vi "main(Test DQMH modules).vi"() -> ()   [LabVIEW 2018, in "Application.lvlib"]
uses:
  Application.lvlib
  eMIC response.ctl
  type defs/HW config.ctl
  eMICs Cluster.ctl
  SubVIs/App state data.ctl
  SubVIs/Trigger cluster.ctl
  SubVIs/FGV DRV data.ctl
  type defs/DMM all config cluster.ctl
  type defs/DMM config cluster.ctl
  SubVIs/DUT data Mode.ctl
  Instrument Drivers/LV_driver_MBrelay/type defs/FGV enum.ctl
  SubVIs/Step data.ctl
  DRV cluster 2.ctl
  <vilib>/ErrorRing/Error Ring.xnode
  Switches Module/MB switches Module.lvlib
  MB 01 switches Module/MB 01 switches Module.lvlib
  DMM Module/DMM Module.lvlib
  v2_CE14/CE14_v2.lvlib
  Instrument Drivers/LV_driver_MBrelay/MB Relay.lvlib
panel:
  out "List of Actions":string[](array[string])
  out "1":u32(colorbox)
  out "elapsed Time":string
  out "#DRV":string
  out "Report file Name":string
  in  "RE_Test":bool caption="Again"
  in  "wait for (ms)":u32=3000
  in  "Log report":bool
  in  "DRV number":u8=1 max=60
  in  "Test Single DRV":bool
  out "DUT Name":string
  out "SAP ID":string
  out "Progress Status":string
  in  "Auto/Man":bool
  out "DC Measure Completed":bool caption="DC Completed"
  in  "Test Channel 10":bool
  in  "Test Channel 9":bool
  in  "Test Channel 8":bool
  in  "Test Channel 7":bool
  in  "Test Channel 6":bool
  in  "Test Channel 5":bool
  in  "Test Channel 4":bool
  in  "Test Channel 3":bool
  in  "Test Channel 2":bool
  in  "Test Channel 1":bool
  in  "Shorted Circuits Test":bool
  out "CE14  Module did it":bool[](array[boolean])
  out "Inst. 9":bool
  in  "Exit":bool
  out "Inst. 8":bool
  out "Inst. 7":bool
  out "Inst. 6":bool
  out "Inst. 5":bool
  out "Inst. 4":bool
  out "Inst. 3":bool
  out "Inst. 2":bool
  out "Inst. 1":bool
  out "new Trigger?":bool
  out "last Trigger?":bool
  out "error out":errorcluster
  out "State log":string
  out "AC  Completed":bool caption="AC Completed"
  in  "Select CE14 eMIC Module Instance":i32(ring)=-1 items=["All"=-1, "1"=1, "2"=2, "3"=3, "4"=4, "5"=5, "6"=6]
  out "New board?":bool
  in  "Test":bool caption="Again"
  out "DRV 61":u32(colorbox)
  in  "Settings":bool
  in  "VIEW":bool caption="Again"
  out "DRV 60":u32(colorbox) caption="60"
  out "DRV 59":u32(colorbox) caption="59"
  out "DRV 58":u32(colorbox) caption="58"
  out "DRV 57":u32(colorbox) caption="57"
  out "DRV 56":u32(colorbox) caption="56"
  out "DRV 55":u32(colorbox) caption="55"
  out "DRV 54":u32(colorbox) caption="54"
  out "DRV 53":u32(colorbox) caption="53"
  out "DRV 52":u32(colorbox) caption="52"
  out "DRV 51":u32(colorbox) caption="51"
  out "DRV 50":u32(colorbox) caption="50"
  out "DRV 49":u32(colorbox) caption="49"
  out "DRV 48":u32(colorbox) caption="48"
  out "DRV 47":u32(colorbox) caption="47"
  out "DRV 46":u32(colorbox) caption="46"
  out "DRV 45":u32(colorbox) caption="45"
  out "DRV 44":u32(colorbox) caption="44"
  out "DRV 43":u32(colorbox) caption="43"
  out "DRV 42":u32(colorbox) caption="42"
  out "DRV 41":u32(colorbox) caption="41"
  out "DRV 40":u32(colorbox) caption="40"
  out "DRV 39":u32(colorbox) caption="39"
  out "DRV 38":u32(colorbox) caption="38"
  out "DRV 37":u32(colorbox) caption="37"
  out "DRV 36":u32(colorbox) caption="36"
  out "DRV 35":u32(colorbox) caption="35"
  out "DRV 34":u32(colorbox) caption="34"
  out "DRV 33":u32(colorbox) caption="33"
  out "DRV 32":u32(colorbox) caption="32"
  out "DRV 31":u32(colorbox) caption="31"
  out "DRV 30":u32(colorbox) caption="30"
  out "DRV 29":u32(colorbox) caption="29"
  out "DRV 28":u32(colorbox) caption="28"
  out "DRV 27":u32(colorbox) caption="27"
  out "DRV 26":u32(colorbox) caption="26"
  out "DRV 25":u32(colorbox) caption="25"
  out "DRV 24":u32(colorbox) caption="24"
  out "DRV 23":u32(colorbox) caption="23"
  out "DRV 22":u32(colorbox) caption="22"
  out "DRV 21":u32(colorbox) caption="21"
  out "DRV 20":u32(colorbox) caption="20"
  out "DRV 19":u32(colorbox) caption="19"
  out "DRV 18":u32(colorbox) caption="18"
  out "DRV 17":u32(colorbox) caption="17"
  out "DRV 16":u32(colorbox) caption="16"
  out "DRV 15":u32(colorbox) caption="15"
  out "DRV 14":u32(colorbox) caption="14"
  out "DRV 13":u32(colorbox) caption="13"
  out "DRV 12":u32(colorbox) caption="12"
  out "DRV 11":u32(colorbox) caption="11"
  out "DRV 10":u32(colorbox) caption="10"
  out "DRV 9":u32(colorbox) caption="9"
  out "DRV 8":u32(colorbox) caption="8"
  out "DRV 7":u32(colorbox) caption="7"
  out "DRV 6":u32(colorbox) caption="6"
  out "DRV 5":u32(colorbox) caption="5"
  out "DRV 4":u32(colorbox) caption="4"
  out "DRV 3":u32(colorbox) caption="3"
  out "DRV 2":u32(colorbox) caption="2"
  out "DRV 1":u32(colorbox) caption="1"
  out "version":string caption="Version"
  out "Module ID":i32
  in  "Tab Control":T1(tab)
  out "Short DRV":bool[][](array[boolean])
  in  "Mux 10-1":bool
  in  "mux 6-1":bool
  in  "Read Optos":bool
  in  "Select DMM's Current Input":bool
  in  "mux2-1(DMM I) encode":enum16{"DMM I (0.5)", "DMM I (12)"}(ring)
  in  "mux 6-1 data":T2(ring)
  in  "mux 10-1 data":T3(ring)
  in  "set value":bool
  in  "Set trigger value":bool
  out "trigger Value":bool
  in  "Read trigger":bool
  in  "Reset JIG":bool
  in  "eMIC":bool
  in  "DEMUX 1-10":bool
  in  "TurnON/OFF +5V":bool
  in  "5V Value":bool
  in  "demux1_10(x6)_encode":T4(ring)
  in  "eMIC 6 values":bool[](array[boolean])=[FALSE, FALSE, FALSE, FALSE, FALSE, FALSE]
  in  "DMM query":bool
  in  "connect DMM":bool
  in  "DMM read dual value":bool
  in  "config DMM":bool
  in  "Detector Rate":u8(ring)=2 items=["SLOW", "MID", "FAST"]
  in  "DCI range":dbl=0.5
  in  "DCV range":dbl=1000.0
  out "DCV(Volts)":dbl
  out "DCI(mA)":dbl
  out "DMM func?":string
  out "DMM range?":string
  in  "request AC-all":bool
  in  "Open COM eMIC":bool
  in  "check connected":bool
  out "eMIC 1":T5
  out "eMIC 2":T5
  out "eMIC 3":T5
  out "eMIC 4":T5
  out "eMIC 5":T5
  out "eMIC 6":T5
  out "EMIC connected":bool[](array[boolean])
  out "AC switches Module":bool
  out "DC Measure Module":bool
  out "DC Switches Module":bool
  out "AC Measure Module":bool
  # "HV-60D: ON-LINE TESTER FOR LED POWER DRIVER"
  # "60"
  # "6"
  # "12"
  # "18"
  # "24"
  # "30"
  # "36"
  # "42"
  # "48"
  # "54"
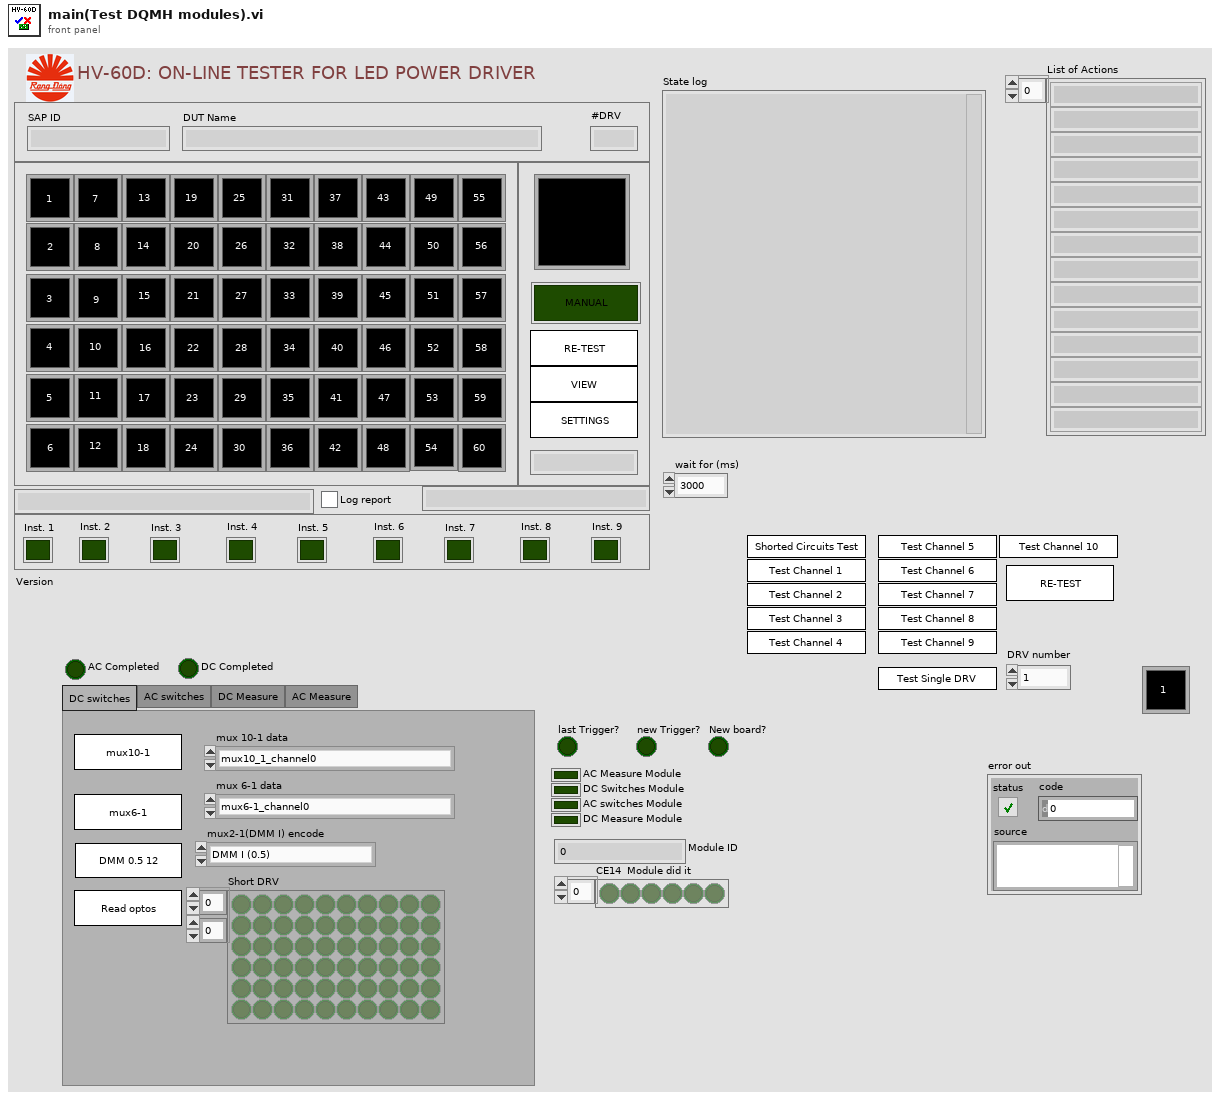
[diagram p1: front panel]
types:
  T1 = enum32{"DC switches", "AC switches", "DC Measure", "AC Measure"}
  T2 = enum16{"mux6-1_channel0", "mux6_1_channel1_0", "mux6_1_channel1_1", "mux6-1_channel1_2", "mux6_1_channel1_3", "mux6_1_channel2_0", "mux6_1_channel2_1", "mux6_1_channel2_2", "mux6_1_channel2_3", "mux6_1_channel3_0", "mux6_1_channel3_1", "mux6_1_channel3_2", "mux6_1_channel3_3", "mux6_1_channel4_0", "mux6_1_channel4_1", "mux6_1_channel4_2", "mux6_1_channel4_3", "mux6_1_channel5_0", "mux6_1_channel5_1", "mux6_1_channel5_2", "mux6_1_channel5_3", "mux6_1_channel6_0", "mux6_1_channel6_1", "mux6_1_channel6_2", "mux6_1_channel6_3"}
  T3 = enum16{"mux10_1_channel0", "mux10_1_channel1", "mux10_1_channel2", "mux10_1_channel3", "mux10_1_channel4", "mux10_1_channel5", "mux10_1_channel6", "mux10_1_channel7", "mux10_1_channel8", "mux10_1_channel9", "mux10_1_channel10"}
  T4 = enum16{"demux1_10_channel0", "demux1_10_channel1", "demux1_10_channel2", "demux1_10_channel3", "demux1_10_channel4", "demux1_10_channel5", "demux1_10_channel6", "demux1_10_channel7", "demux1_10_channel8", "demux1_10_channel9", "demux1_10_channel10"}
  T5 = typedef "Application.lvlib/eMIC response.ctl" = cluster{"ACV":dbl, "ACI":dbl, "pF":dbl, "kW":dbl, "Freq":dbl, "kvar":dbl}
  T6 = typedef "Application.lvlib/eMICs Cluster.ctl" = cluster{"eMIC 1":T5, "eMIC 2":T5, "eMIC 3":T5, "eMIC 4":T5, "eMIC 5":T5, "eMIC 6":T5}
  T7 = typedef "Application.lvlib/HW config.ctl" = cluster{"DMM":string, "mux":string, "demux":string, "eMIC1":string, "eMIC2":string, "eMIC3":string, "eMIC4":string, "eMIC5":string, "eMIC6":string}
  T8 = typedef "Application.lvlib/Trigger cluster.ctl" = cluster{"new board?":bool, "new trigger":bool, "last trigger":bool}
  T9 = typedef "Application.lvlib/App state data.ctl" = cluster{"command":string, "data":variant}
  T10 = typedef "CE14_v2.lvlib/Broadcast Events--cluster.ctl" = cluster{"Module Did Init":refnum<user-event>, "Status Updated":refnum<user-event>, "Error Reported":refnum<user-event>, "Module Did Stop":refnum<user-event>, "Update Module Execution Status":refnum<user-event>, "CE14 response data":refnum<user-event>}
  T11 = typedef "MB switches Module.lvlib/Broadcast Events--cluster.ctl" = cluster{"Module Did Init":refnum<user-event>, "Status Updated":refnum<user-event>, "Error Reported":refnum<user-event>, "Module Did Stop":refnum<user-event>, "Update Module Execution Status":refnum<user-event>}
  T12 = typedef "MB 01 switches Module.lvlib/Broadcast Events--cluster.ctl" = cluster{"Module Did Init":refnum<user-event>, "Status Updated":refnum<user-event>, "Error Reported":refnum<user-event>, "Module Did Stop":refnum<user-event>, "Update Module Execution Status":refnum<user-event>}
  T13 = typedef "DMM Module.lvlib/Broadcast Events--cluster.ctl" = cluster{"Module Did Init":refnum<user-event>, "Status Updated":refnum<user-event>, "Error Reported":refnum<user-event>, "Module Did Stop":refnum<user-event>, "Update Module Execution Status":refnum<user-event>}
  T14 = enum16{"open", "replace", "create", "open or create", "replace or create", "replace or create with confirmation"}
  T15 = typedef "Application.lvlib/DRV cluster 2.ctl" = cluster{"Shorted Circuit":bool, "AC voltage(volts)":dbl, "AC Current (mA)":dbl, "AC kW (W)":dbl, "AC pF ":dbl, "DC Voltage (Volts)":dbl, "DC Current (mA)":dbl, "DC kW (W)":dbl, "DRV Fail/Pass (T)":bool, "efficient (%)":dbl}
  T16 = typedef "Application.lvlib/DRV stand.ctl" = cluster{"SAP ID":string, "Name":string, "AC characteristics":cluster{"Voltage":cluster{"Min":dbl, "Max":dbl}, "Current":cluster{"Min":dbl, "Max":dbl}, "kW":cluster{"Min":dbl, "Max":dbl}, "PF":cluster{"Min":dbl, "Max":dbl}}, "DC characteristics":cluster{"Voltage":cluster{"Min":dbl, "Max":dbl}, "Current":cluster{"Min":dbl, "Max":dbl}, "Effect":cluster{"Min":dbl, "Max":dbl}}, "Sub-Test":cluster{"ACV":bool, "ACI":bool, "kW":bool, "PF":bool, "DCV":bool, "DCI":bool, "efficiency":bool}}
  T17 = enum32{"Invalid", "Standard", "Closed", "Hidden", "Minimized", "Maximized"}
  T18 = typedef "Application.lvlib/FGV DRV data.ctl" = enum16{"Init", "Write", "Read", "Process"}
  T19 = typedef "Application.lvlib/DMM all config cluster.ctl" = cluster{"DMM config cluster":T20, "mux2-1(DMM I) encode":enum16{"DMM I (0.5)", "DMM I (12)"}}
  T20 = typedef "Application.lvlib/DMM config cluster.ctl" = cluster{"DCV range":dbl, "DCI range":dbl, "Detector Rate":u8}
  T21 = typedef "Application.lvlib/DUT data Mode.ctl" = enum16{"range Limit", "Short Circuits", "AC parameter", "AC parameter 1", "DC parameter"}
  T22 = typedef "MB Relay.lvlib/FGV enum.ctl" = enum16{"Write", "Init FGV", "Read", "All OFF", "All ON"}
  T23 = typedef "CE14_eMIC.lvlib/CE14.data.ctl" = cluster{"string":string, "float":dbl, "Name":string}
  T24 = typedef "Application.lvlib/Step data.ctl" = cluster{"command":string, "Data":variant}
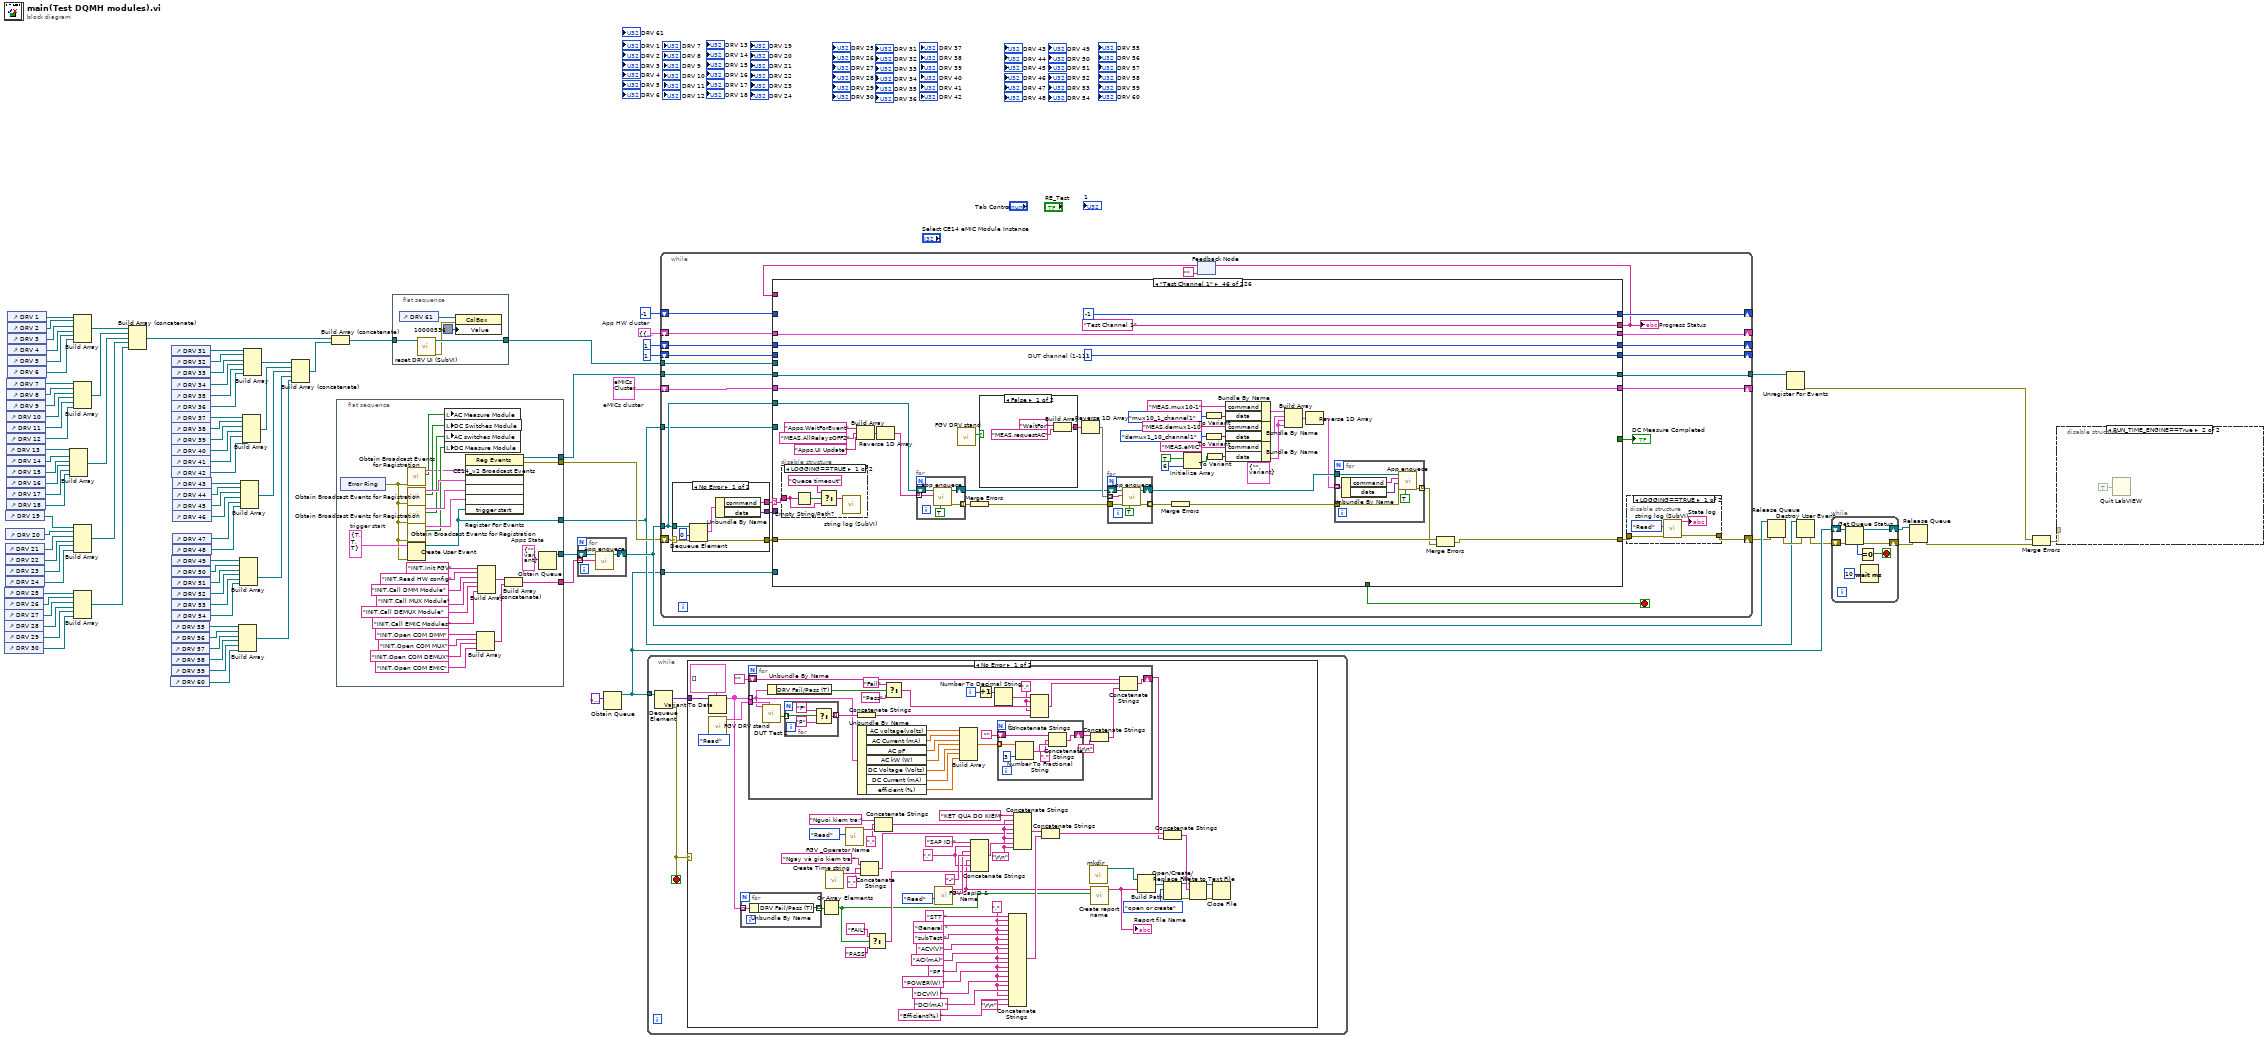
[diagram p0: block diagram]
diagram:
  w88 = T6 {"eMIC 1"={"ACV"=0.0, "ACI"=0.0, "pF"=0.0, "kW"=0.0, "Freq"=0.0, "kvar"=0.0}, "eMIC 2"={"ACV"=0.0, "ACI"=0.0, "pF"=0.0, "kW"=0.0, "Freq"=0.0, "kvar"=0.0}, "eMIC 3"={"ACV"=0.0, "ACI"=0.0, "pF"=0.0, "kW"=0.0, "Freq"=0.0, "kvar"=0.0}, "eMIC 4"={"ACV"=0.0, "ACI"=0.0, "pF"=0.0, "kW"=0.0, "Freq"=0.0, "kvar"=0.0}, "eMIC 5"={"ACV"=0.0, "ACI"=0.0, "pF"=0.0, "kW"=0.0, "Freq"=0.0, "kvar"=0.0}, "eMIC 6"={"ACV"=0.0, "ACI"=0.0, "pF"=0.0, "kW"=0.0, "Freq"=0.0, "kvar"=0.0}}  # eMICs cluster
  w93 = cluster{"HW config 2":T7} {"HW config 2"={"DMM"="COM15", "mux"="COM11", "demux"="COM16", "eMIC1"="COM13", "eMIC2"="COM6", "eMIC3"="COM9", "eMIC4"="COM10", "eMIC5"="COM12", "eMIC6"="COM11"}}  # App HW cluster
  n1 = control-ref of="DRV 25"() -> (w58:refnum<vi>)
  n2 = control-ref of="DRV 26"() -> (w59:refnum<vi>)
  n3 = control-ref of="DRV 27"() -> (w60:refnum<vi>)
  n4 = control-ref of="DRV 28"() -> (w61:refnum<vi>)
  n5 = control-ref of="DRV 29"() -> (w62:refnum<vi>)
  n6 = control-ref of="DRV 30"() -> (w63:refnum<vi>)
  n7 = control-ref of="DRV 21"() -> (w67:refnum<vi>)
  n8 = control-ref of="DRV 22"() -> (w66:refnum<vi>)
  n9 = control-ref of="DRV 23"() -> (w65:refnum<vi>)
  n10 = control-ref of="DRV 24"() -> (w64:refnum<vi>)
  n11 = control-ref of="DRV 19"() -> (w69:refnum<vi>)
  n12 = control-ref of="DRV 20"() -> (w68:refnum<vi>)
  n13 = control-ref of="DRV 13"() -> (w75:refnum<vi>)
  n14 = control-ref of="DRV 7"() -> (w81:refnum<vi>)
  n15 = control-ref of="DRV 8"() -> (w80:refnum<vi>)
  n16 = control-ref of="DRV 9"() -> (w79:refnum<vi>)
  n17 = control-ref of="DRV 10"() -> (w78:refnum<vi>)
  n18 = control-ref of="DRV 11"() -> (w77:refnum<vi>)
  n19 = control-ref of="DRV 12"() -> (w76:refnum<vi>)
  n20 = control-ref of="DRV 14"() -> (w74:refnum<vi>)
  n21 = control-ref of="DRV 15"() -> (w73:refnum<vi>)
  n22 = control-ref of="DRV 16"() -> (w72:refnum<vi>)
  n23 = control-ref of="DRV 17"() -> (w71:refnum<vi>)
  n24 = control-ref of="DRV 18"() -> (w70:refnum<vi>)
  n25 = control-ref of="DRV 1"() -> (w87:refnum<vi>)
  n26 = control-ref of="DRV 2"() -> (w86:refnum<vi>)
  n27 = control-ref of="DRV 3"() -> (w85:refnum<vi>)
  n28 = control-ref of="DRV 4"() -> (w84:refnum<vi>)
  n29 = control-ref of="DRV 5"() -> (w83:refnum<vi>)
  n30 = control-ref of="DRV 6"() -> (w82:refnum<vi>)
  n31 = Build Array(w75, w74, w73, w72, w71, w70) -> (w55:refnum<vi>[])
  n32 = Build Array(w87, w86, w85, w84, w83, w82) -> (w57:refnum<vi>[])
  n33 = Build Array(w69, w68, w67, w66, w65, w64) -> (w54:refnum<vi>[])
  n34 = Build Array(w58, w59, w60, w61, w62, w63) -> (w53:refnum<vi>[])
  n35 = Build Array(w81, w80, w79, w78, w77, w76) -> (w56:refnum<vi>[])
  n36 = Build Array (concatenate)(w57, w56, w55, w54, w53) -> (w17:refnum<vi>[])
  n37 = control-ref of="DRV 60"() -> (w28:refnum<vi>)
  n38 = control-ref of="DRV 55"() -> (w23:refnum<vi>)
  n39 = control-ref of="DRV 56"() -> (w24:refnum<vi>)
  n40 = control-ref of="DRV 57"() -> (w25:refnum<vi>)
  n41 = control-ref of="DRV 58"() -> (w26:refnum<vi>)
  n42 = control-ref of="DRV 59"() -> (w27:refnum<vi>)
  n43 = control-ref of="DRV 31"() -> (w47:refnum<vi>)
  n44 = control-ref of="DRV 32"() -> (w48:refnum<vi>)
  n45 = control-ref of="DRV 33"() -> (w49:refnum<vi>)
  n46 = control-ref of="DRV 34"() -> (w50:refnum<vi>)
  n47 = control-ref of="DRV 35"() -> (w51:refnum<vi>)
  n48 = control-ref of="DRV 36"() -> (w52:refnum<vi>)
  n49 = control-ref of="DRV 37"() -> (w46:refnum<vi>)
  n50 = control-ref of="DRV 38"() -> (w45:refnum<vi>)
  n51 = control-ref of="DRV 39"() -> (w44:refnum<vi>)
  n52 = control-ref of="DRV 40"() -> (w43:refnum<vi>)
  n53 = control-ref of="DRV 41"() -> (w42:refnum<vi>)
  n54 = control-ref of="DRV 42"() -> (w41:refnum<vi>)
  n55 = control-ref of="DRV 49"() -> (w34:refnum<vi>)
  n56 = control-ref of="DRV 50"() -> (w33:refnum<vi>)
  n57 = control-ref of="DRV 51"() -> (w32:refnum<vi>)
  n58 = control-ref of="DRV 52"() -> (w31:refnum<vi>)
  n59 = control-ref of="DRV 53"() -> (w30:refnum<vi>)
  n60 = control-ref of="DRV 54"() -> (w29:refnum<vi>)
  n61 = control-ref of="DRV 43"() -> (w35:refnum<vi>)
  n62 = control-ref of="DRV 44"() -> (w36:refnum<vi>)
  n63 = control-ref of="DRV 45"() -> (w37:refnum<vi>)
  n64 = control-ref of="DRV 46"() -> (w38:refnum<vi>)
  n65 = control-ref of="DRV 47"() -> (w39:refnum<vi>)
  n66 = control-ref of="DRV 48"() -> (w40:refnum<vi>)
  n67 = Build Array(w23, w24, w25, w26, w27, w28) -> (w18:refnum<vi>[])
  n68 = Build Array(w34, w33, w32, w31, w30, w29) -> (w19:refnum<vi>[])
  n69 = Build Array(w35, w36, w37, w38, w39, w40) -> (w20:refnum<vi>[])
  n70 = Build Array(w46, w45, w44, w43, w42, w41) -> (w21:refnum<vi>[])
  n71 = Build Array(w47, w48, w49, w50, w51, w52) -> (w22:refnum<vi>[])
  n72 = Build Array (concatenate)(w22, w21, w20, w19, w18) -> (w16:refnum<vi>[])
  n73 = Build Array (concatenate)(w17, w16) -> (w14:refnum<vi>[])
  n74 = flat-sequence {
    tunnel: [w118] -> w95
    tunnel: [w117] -> w92
    tunnel: [w116] -> w91
    tunnel: [w115] -> w15
    tunnel: [w110] -> w7
    frame #0 {
      w111 = T8 {"new board?"=TRUE, "new trigger"=TRUE, "last trigger"=TRUE}  # trigger start
      w112 = T9 {"command"="", "data"=variant}  # Apps State
      n75 = xnode "Error Ring"() -> ("error out"=w109:errorcluster)
      n76 = call "Obtain Broadcast Events for Registration.vi"("error in (no error)"=w109) -> ("Already running?"=w113:bool, "CE14_v2 Broadcast Events"=w114:T10)  [unwired: 8 in, 1 out]
      n77 = call "Obtain Broadcast Events for Registration.vi"("error in (no error)"=w109) -> ("Already running?"=w121:bool, "Switches Module Broadcast Events"=w124:T11)  [unwired: 8 in, 1 out]
      n78 = call "Obtain Broadcast Events for Registration.vi"("error in (no error)"=w109) -> ("Already running?"=w120:bool, "MB 01 switches Module Broadcast Events"=w123:T12)  [unwired: 8 in, 1 out]
      n79 = call "Obtain Broadcast Events for Registration.vi"("error in (no error)"=w109) -> ("Already running?"=w119:bool, "DMM Module Broadcast Events"=w122:T13)  [unwired: 8 in, 1 out]
      n80 = Create User Event(user event datatype=w111, error in=w109) -> (user event=w110:refnum<user-event>)  [unwired: 1 out]
      n81 = local write "AC Measure Module"(w113) -> ()
      n82 = local write "DC Switches Module"(w121) -> ()
      n83 = local write "AC switches Module"(w120) -> ()
      n84 = local write "DC Measure Module"(w119) -> ()
      n85 = register-events(w114, w124, w123, w122, w110) -> (reference out=w118:refnum<event-registration>, error out=w115:errorcluster)  [unwired: 2 in]
      n86 = Build Array("INIT.Open COM DMM", "INIT.Open COM MUX", "INIT.Open COM DEMUX", "INIT.Open COM EMIC") -> (w106:string[])
      n87 = Build Array("INIT.Init FGV", "INIT.Read HW config", "INIT.Call DMM Module", "INIT.Call MUX Module", "INIT.Call DEMUX Module", "INIT.Call EMIC Modules") -> (w107:string[])
      n88 = Build Array (concatenate)(w107, w106) -> (w116:string[])
      n89 = Obtain Queue(element data type=w112) -> (queue out=w117:refnum<queue>)  [unwired: 4 in, 2 out]
    }
  }
  n90 = flat-sequence {
    tunnel: w14 -> [w130]
    tunnel: [w129] -> w13
    frame #0 {
      n91 = control-ref of="DRV 61"() -> (w126:refnum<vi>)
      n92 = call "reset DRV UI (SubVI).vi"("Ref  in"=w130) -> ("error out"=w127:errorcluster, "Ref out"=w129:refnum<vi>[])  [unwired: 9 in]
      n93 = property class="ColBox"(reference=w126, error in=w127, "Value"=u32 10000536 ("DRV 1")) -> ()  [unwired: 2 out]
    }
  }
  n94 = for {
    tunnel: w91 -> [w133] mode=indexing
    shift-right: [w131] -> w90
    shift-left: w92 -> [w132]
    n95 = call "App enquece.vi"("command"=w133, "queue in"=w132) -> ("Queue out"=w131:refnum<queue>)  [unwired: 8 in, 1 out]
  }
  n96 = Obtain Queue(element data type=variant) -> (queue out=w5:refnum<queue>)  [unwired: 4 in, 2 out]
  n97 = while {
    tunnel: w5 -> [w136]
    stop <- w134 stop-if-true
    n98 = Dequeue Element(queue=w136) -> (element=w135:variant, error out=w134:errorcluster)  [unwired: 2 in, 2 out]
    n99 = case shown="No Error" w134 {
      tunnel: w135 -> [w189 _]
      frame No Error {
        w156 = ","
        w140 = ","
        w163 = "\r\n"
        n100 = Variant To Data(type=T15[] [] ("60 DRV data"), Variant=w189) -> (data=w144:T15[])  [unwired: 1 in, 1 out]
        n101 = call "FGV DRV stand.vi"("Enum(read)"=enum16{"Write", "Read"}."Read" ("Enum 2")) -> ("DRV stand out"=w187:T16)  [unwired: 9 in, 1 out]
        n102 = for {
          tunnel: w144 -> [w192] mode=indexing
          tunnel: [w191] -> w141 mode=indexing
          n103 = Unbundle By Name(w192) -> ("DRV Fail/Pass (T)"=w191:bool)
        }
        n104 = for {
          tunnel: w144 -> [w209] mode=indexing
          tunnel: w187 -> [w220]
          shift-right: [w197] -> w165
          shift-left: "" -> [w196]
          i -> [w214]
          w193 = ","
          n105 = call "DUT Test 2.vi"("DRV stand"=w220, "DRV data"=w209) -> ("actual subtest"=w216:bool[])  [unwired: 6 in, 3 out]
          n106 = Unbundle By Name(w209) -> ("DRV Fail/Pass (T)"=w219:bool)
          n107 = for {
            tunnel: w216 -> [w229] mode=indexing
            tunnel: [w228] -> w215 mode=indexing
            n108 = Select(t="F", s=w229, f="P") -> (s? t:f=w228:string)
          }
          n109 = Concatenate Strings(w215) -> (w210:string)
          n110 = Unbundle By Name(w209) -> ("AC voltage(volts)"=w208:dbl, "AC Current (mA)"=w207:dbl, "AC pF"=w206:dbl, "AC kW (W)"=w205:dbl, "DC Voltage (Volts)"=w204:dbl, "DC Current (mA)"=w203:dbl, "efficient (%)"=w202:dbl)
          n111 = Select(t="Fail", s=w219, f="Pass") -> (s? t:f=w211:string)
          n112 = Build Array(w208, w207, w206, w205, w204, w203, w202) -> (w201:dbl[])
          n113 = Increment(x=w214) -> (x+1=w213:i32)
          n114 = Number To Decimal String(number=w213) -> (decimal integer string=w212:string)  [unwired: 1 in]
          n115 = for {
            tunnel: w201 -> [w226] mode=indexing
            shift-right: [w223] -> w199
            shift-left: "" -> [w224]
            n116 = Number To Fractional String(number=w226, precision (6)=i16 3) -> (F-format string=w222:string)  [unwired: 2 in]
            n117 = Concatenate Strings(w224, ",", w222) -> (w223:string)
          }
          n118 = Concatenate Strings(w212, w193, w211, w193, w210) -> (w195:string)
          n119 = Concatenate Strings(w199, "\r\n") -> (w194:string)
          n120 = Concatenate Strings(w196, w195, w194) -> (w197:string)
        }
        n121 = Or Array Elements(Boolean array=w141) -> (logical OR=w137:bool)
        n122 = call "Create Time string.vi"() -> ("Timestr"=w161:string)  [unwired: 10 in, 1 out]
        n123 = call "FGV _Operator Name.vi"("Enum"=enum16{"Write", "Read"}."Read") -> ("Operator Name out"=w185:string)  [unwired: 10 in]
        n124 = Concatenate Strings("Ngay và gio kiem tra:", ",", w161) -> (w160:string)
        n125 = Select(t="FAIL", s=w137, f="PASS") -> (s? t:f=w139:string)
        n126 = Concatenate Strings("Nguoi kiem tra:", ",", w185) -> (w186:string)
        n127 = call "FGV SapID & Name.vi"("Enum"=enum16{"Read", "Write"}."Read") -> ("Name out"=w147:string, "SAP ID out"=w138:string)  [unwired: 9 in]
        n128 = Concatenate Strings("SAP ID:", w140, w147, "-", w138, w140, w139) -> (w164:string)
        n129 = Concatenate Strings("STT ", w156, "General ", w156, "subTest ", w156, "ACV(V)", w156, "ACI(mA)", w156, "PF ", w156, "POWER(W) ", w156, "DCV(V) ", w156, "DCI(mA) ", w156, "Efficient(%) ", "\r\n") -> (w168:string)
        n130 = Concatenate Strings("KET QUA DO KIEM" ("string"), w163, w186, w163, w160, w163, w164, w163) -> (w167:string)
        n131 = Concatenate Strings(w167, w168) -> (w166:string)
        n132 = call "mkdir.vi"() -> ("created path"=w155:path)  [unwired: 10 in, 1 out]
        n133 = call "Create report name.vi"("PCB Pass/Fail"=w137, "SAP ID"=w138) -> ("filename"=w145:string)  [unwired: 8 in, 1 out]
        "Report file Name" <- w145
        n134 = Build Path(base path=w155, name or relative path=w145) -> (appended path=w154:path)
        n135 = Concatenate Strings(w166, w165) -> (w152:string)
        n136 = Open/Create/Replace File(file path (use dialog)=w154, operation (0:open)=T14."open or create") -> (refnum out=w151:refnum<file>, error out=w150:errorcluster)  [unwired: 4 in, 1 out]
        n137 = Write to Text File(file (use dialog)=w151, text=w152, error in=w150) -> (refnum out=w148:refnum<file>, error out=w149:errorcluster)  [unwired: 1 in, 1 out]
        n138 = Close File(refnum=w148, error in=w149) -> ()  [unwired: 2 out]
      }
      frame Error {
      }
    }
  }
  n139 = while {
    shift-right: [w235] -> w89
    shift-left: w15 -> [w257]
    shift-right: [w255] -> _
    shift-left: -1 -> [w254]
    tunnel: w95 -> [w253]
    tunnel: [w252] -> w94
    shift-right: [w250] -> _
    shift-left: w93 -> [w251]
    tunnel: w90 -> [w239]
    shift-right: [w248] -> _
    shift-left: w88 -> [w247]
    tunnel: w13 -> [w245]
    shift-right: [w244] -> _
    shift-left: 1 ("DUT channel (1-11)") -> [w243]
    shift-right: [w242] -> _
    shift-left: 1 ("DUT index(0-59)") -> [w241]
    tunnel: w7 -> [w238]
    tunnel: w5 -> [w231]
    stop <- w246 stop-if-true
    n140 = case shown="No Error" w257 {
      selector: w257 -> [w268 w269]
      tunnel: [w266 "Apps.Error Handler"] -> w240
      tunnel: [w267 w269] -> w256
      tunnel: [w265 _] -> w249
      tunnel: w239 -> [w264 _]
      frame No Error {
        n141 = Dequeue Element(queue=w264, timeout in ms (-1)=0, error in (no error)=w268) -> (element=w263:T9, error out=w267:errorcluster)  [unwired: 2 out]
        n142 = Unbundle By Name(w263) -> ("command"=w266:string, "data"=w265:variant)
      }
      frame Error {
      }
    }
    n143 = feedback #1("") -> (w233:string)
    n144 = case shown="\"Test Channel 1\"" w240 {
      selector: w240 -> [w279 _ _ w1255 w1274 w1411 w1441 w1487 _ _ _ _ _ _ _ _ w1625 w1647 _ w1705 w1762 w1799 w1821 w1844 w1867 w1900 w1918 w1936 w1954 w1987 w2014 w2039 w2067 w2100 w2117 w2141 w2174 w2190 w2214 w2245 w2273 w2306 w2349 w2385 w2428 w2493 w2568 w2644 w2718 w2793 w2868 w2929 w3032 w3108 w3183 w3266 w3348 w3430 w3512 w3594 w3676 w3758 w3840 w3922 w4004 w4086 w4169 w4252 w4335 w4418 w4501 w4566 w4685 w4768 w4851 w4934 w5018 w5102 w5186 w5270 w5354 w5438 w5522 w5606 w5690 w5774 w5859 w5944 w6029 w6114 w6199 w6284 w6369 w6454 w6539 w6624 w6710 w6796 w6882 w6968 w7054 w7140 w7226 w7312 w7398 w7448 w7488 w7528 w7569 w7610 w7650 w7692 w7733 w7774 w7815 w7856 w7897 w7938 w7979 w8020 w8062 w8102 w8142 w8184 w8225 w8267 w8307 w8349 w8389 w8430 w8472 w8512 w8553 w8594 w8635 w8676 w8717 w8758 w8800 w8840 w8881 w8922 w8964 w9005 w9045 w9086 w9127 w9168 w9209 w9250 w9291 w9332 w9373 w9414 w9455 w9496 w9537 w9578 w9619 w9659 w9701 w9742 w9783 w9824 w9865 _ w9916 w10014 w10112 w10210 w10309 w10408 w10507 w10606 w10705 w10804 w10903 w11002 w11101 w11200 w11299 w11398 w11497 w11596 w11695 w11794 w11893 w11992 w12091 w12190 w12289 w12388 w12487 w12586 w12685 w12784 w12883 w12982 w13081 w13180 w13279 w13378 w13477 w13576 w13675 w13774 w13873 w13972 w14071 w14170 w14269 w14368 w14467 w14566 w14665 w14764 w14863 w14962 w15061 w15160 w15259 w15358 w15457 w15556 w15655 w15754]
      tunnel: w256 -> [w285 w1241 w1243 w1256 w1281 w1413 w1454 w1495 w1520 w1528 w1539 w1550 w1565 w1580 w1595 w1610 w1633 w1661 w1685 w1717 w1763 w1800 w1822 w1845 w1868 w1901 w1919 w1937 w1955 w1971 w2015 w2040 w2068 w2085 w2120 w2140 w2175 w2191 w2215 w2246 w2277 w2307 w2352 w2386 w2416 w2495 w2570 w2609 w2720 w2795 w2870 w2931 w3034 w3110 w3185 w3268 w3350 w3432 w3514 w3596 w3678 w3760 w3842 w3924 w4006 w4088 w4171 w4254 w4337 w4420 w4503 w4568 w4687 w4770 w4853 w4936 w5020 w5104 w5188 w5272 w5356 w5440 w5524 w5608 w5692 w5776 w5861 w5946 w6031 w6116 w6201 w6286 w6371 w6456 w6541 w6626 w6712 w6798 w6884 w6970 w7056 w7142 w7228 w7314 w7400 w7451 w7493 w7533 w7574 w7615 w7656 w7697 w7738 w7779 w7820 w7861 w7902 w7943 w7984 w8025 w8067 w8107 w8148 w8189 w8230 w8272 w8312 w8354 w8394 w8435 w8477 w8517 w8558 w8599 w8640 w8681 w8722 w8763 w8805 w8845 w8886 w8927 w8969 w9010 w9050 w9091 w9132 w9173 w9214 w9255 w9296 w9337 w9378 w9419 w9460 w9501 w9542 w9583 w9624 w9665 w9706 w9747 w9788 w9829 w9870 w9908 w9921 w10019 w10117 w10215 w10314 w10413 w10512 w10611 w10710 w10809 w10908 w11007 w11106 w11205 w11304 w11403 w11502 w11601 w11700 w11799 w11898 w11997 w12096 w12195 w12294 w12393 w12492 w12591 w12690 w12789 w12888 w12987 w13086 w13185 w13284 w13383 w13482 w13581 w13680 w13779 w13878 w13977 w14076 w14175 w14274 w14373 w14472 w14571 w14670 w14769 w14868 w14967 w15066 w15165 w15264 w15363 w15462 w15561 w15660 w15759]
      tunnel: [w286 w1241 w1244 w1257 w1282 w1414 w1436 w1486 w1520 w1527 w1538 w1549 w1564 w1579 w1594 w1609 w1634 w1649 w1675 w1708 w1760 w1801 w1823 w1846 w1866 w1899 w1917 w1935 w1953 w1979 w2013 w2037 w2064 w2101 w2119 w2142 w2171 w2195 w2217 w2249 w2275 w2299 w2350 w2384 w2419 w2496 w2571 w2646 w2721 w2796 w2871 w2932 w3035 w3111 w3163 w3269 w3351 w3433 w3515 w3597 w3679 w3761 w3843 w3925 w4007 w4089 w4172 w4255 w4338 w4421 w4504 w4569 w4688 w4771 w4854 w4937 w5021 w5105 w5189 w5273 w5357 w5441 w5525 w5609 w5693 w5777 w5862 w5947 w6032 w6117 w6202 w6287 w6372 w6457 w6542 w6627 w6713 w6799 w6885 w6971 w7057 w7143 w7229 w7315 w7401 w7452 w7482 w7534 w7575 w7616 w7657 w7698 w7739 w7780 w7821 w7862 w7903 w7944 w7985 w8026 w8057 w8108 w8149 w8190 w8231 w8265 w8313 w8347 w8395 w8436 w8470 w8518 w8559 w8600 w8641 w8682 w8723 w8764 w8798 w8846 w8887 w8928 w8962 w8999 w9051 w9092 w9133 w9174 w9215 w9256 w9297 w9338 w9379 w9420 w9461 w9502 w9543 w9584 w9625 w9666 w9707 w9748 w9789 w9830 w9871 w9908 w9919 w10017 w10115 w10213 w10312 w10411 w10510 w10609 w10708 w10807 w10906 w11005 w11104 w11203 w11302 w11401 w11500 w11599 w11698 w11797 w11896 w11995 w12094 w12193 w12292 w12391 w12490 w12589 w12688 w12787 w12886 w12985 w13084 w13183 w13282 w13381 w13480 w13579 w13678 w13777 w13876 w13975 w14074 w14173 w14272 w14371 w14470 w14569 w14668 w14767 w14866 w14965 w15064 w15163 w15262 w15361 w15460 w15559 w15658 w15757] -> w236
      tunnel: [_ _ _ _ _ _ _ _ _ _ _ _ _ _ _ _ TRUE _ _ _ _ _ _ _ _ _ _ _ _ _ _ _ _ _ _ _ _ _ _ _ _ _ _ _ _ _ _ _ _ _ _ _ _ _ _ _ _ _ _ _ _ _ _ _ _ _ _ _ _ _ _ _ _ _ _ _ _ _ _ _ _ _ _ _ _ _ _ _ _ _ _ _ _ _ _ _ _ _ _ _ _ _ _ _ _ _ _ _ _ _ _ _ _ _ _ _ _ _ _ _ _ _ _ _ _ _ _ _ _ _ _ _ _ _ _ _ _ _ _ _ _ _ _ _ _ _ _ _ _ _ _ _ _ _ _ _ _ _ _ _ _ _ _ _ _ _ _ _ _ _ _ _ _ _ _ _ _ _ _ _ _ _ _ _ _ _ _ _ _ _ _ _ _ _ _ _ _ _ _ _ _ _ _ _ _ _ _ _ _ _ _ _ _ _ _ _ _ _ _ _ _ _ _ _ _ _] -> w246
      tunnel: [w290 150 w1253 w1266 w1285 w1417 w1437 w1494 w1519 w1535 w1546 w1557 w1572 w1587 w1602 w1617 w1640 w1660 w1684 w1716 w1770 w1815 w1837 w1859 w1882 w1908 w1926 w1944 w1963 w1994 w2029 -1 w2063 w2092 w2130 w2148 -1 w2202 w2225 w2263 w2283 w2315 w2360 w2391 w2446 -1 -1 -1 -1 -1 -1 -1 -1 -1 -1 -1 -1 -1 -1 -1 -1 -1 -1 -1 -1 -1 -1 -1 -1 -1 -1 -1 -1 -1 -1 -1 -1 -1 -1 -1 -1 -1 -1 -1 -1 -1 -1 -1 -1 -1 -1 -1 -1 -1 -1 -1 -1 -1 -1 -1 -1 -1 -1 -1 -1 w7457 w7498 w7539 w7580 w7621 w7662 w7703 w7744 w7785 w7826 w7867 w7908 w7949 w7990 w8031 w8072 w8113 w8154 w8195 w8236 w8277 w8318 w8359 w8400 w8441 w8482 w8523 w8564 w8605 w8646 w8687 w8728 w8769 w8810 w8851 w8892 w8933 w8974 w9015 w9056 w9097 w9138 w9179 w9220 w9261 w9302 w9343 w9384 w9425 w9466 w9507 w9548 w9589 w9630 w9671 w9712 w9753 w9794 w9835 w9876 w9907 w9926 w10024 w10122 w10220 w10319 w10418 w10517 w10616 w10715 w10814 w10913 w11012 w11111 w11210 w11309 w11408 w11507 w11606 w11705 w11804 w11903 w12002 w12101 w12200 w12299 w12398 w12497 w12596 w12695 w12794 w12893 w12992 w13091 w13190 w13289 w13388 w13487 w13586 w13685 w13784 w13883 w13982 w14081 w14180 w14279 w14378 w14477 w14576 w14675 w14774 w14873 w14972 w15071 w15170 w15269 w15368 w15467 w15566 w15665 w15764] -> w255
      tunnel: w254 -> [w278 _ w1253 w1266 w1285 w1417 w1437 w1494 w1519 w1535 w1546 w1557 w1572 w1587 w1602 w1617 w1640 w1660 w1684 w1716 w1770 w1815 w1837 w1859 w1882 w1908 w1926 w1944 w1963 w1994 w2029 _ w2063 w2091 w2130 w2148 _ w2202 w2225 w2263 w2283 w2315 w2360 w2391 w2446 _ _ _ _ _ _ _ _ _ _ _ _ _ _ _ _ _ _ _ _ _ _ _ _ _ _ _ _ _ _ _ _ _ _ _ _ _ _ _ _ _ _ _ _ _ _ _ _ _ _ _ _ _ _ _ _ _ _ _ _ w7457 w7498 w7539 w7580 w7621 w7662 w7703 w7744 w7785 w7826 w7867 w7908 w7949 w7990 w8031 w8072 w8113 w8154 w8195 w8236 w8277 w8318 w8359 w8400 w8441 w8482 w8523 w8564 w8605 w8646 w8687 w8728 w8769 w8810 w8851 w8892 w8933 w8974 w9015 w9056 w9097 w9138 w9179 w9220 w9261 w9302 w9343 w9384 w9425 w9466 w9507 w9548 w9589 w9630 w9671 w9712 w9753 w9794 w9835 w9876 w9907 w9926 w10024 w10122 w10220 w10319 w10418 w10517 w10616 w10715 w10814 w10913 w11012 w11111 w11210 w11309 w11408 w11507 w11606 w11705 w11804 w11903 w12002 w12101 w12200 w12299 w12398 w12497 w12596 w12695 w12794 w12893 w12992 w13091 w13190 w13289 w13388 w13487 w13586 w13685 w13784 w13883 w13982 w14081 w14180 w14279 w14378 w14477 w14576 w14675 w14774 w14873 w14972 w15071 w15170 w15269 w15368 w15467 w15566 w15665 w15764]
      tunnel: w253 -> [w289 w1240 w1252 w1265 w1284 w1416 w1453 w1493 w1518 w1534 w1545 w1556 w1571 w1586 w1601 w1616 w1639 w1659 w1683 w1715 w1769 w1813 w1835 w1857 w1875 w1907 w1925 w1943 w1962 w1993 w2028 w2047 w2073 w2106 w2129 w2147 w2181 w2201 w2224 w2262 w2282 w2314 w2359 w2390 w2445 w2499 w2575 w2650 w2725 w2800 w2875 w2936 w3039 w3095 w3189 w3273 w3355 w3437 w3519 w3601 w3683 w3765 w3847 w3929 w4011 w4093 w4176 w4259 w4342 w4425 w4508 w4573 w4692 w4775 w4858 w4941 w5025 w5109 w5193 w5277 w5361 w5445 w5529 w5613 w5697 w5781 w5866 w5951 w6036 w6121 w6206 w6291 w6376 w6461 w6546 w6631 w6717 w6803 w6889 w6975 w7061 w7147 w7233 w7319 w7405 w7456 w7497 w7538 w7579 w7620 w7661 w7702 w7743 w7784 w7825 w7866 w7907 w7948 w7989 w8030 w8071 w8112 w8153 w8194 w8235 w8276 w8317 w8358 w8399 w8440 w8481 w8522 w8563 w8604 w8645 w8686 w8727 w8768 w8809 w8850 w8891 w8932 w8973 w9014 w9055 w9096 w9137 w9178 w9219 w9260 w9301 w9342 w9383 w9424 w9465 w9506 w9547 w9588 w9629 w9670 w9711 w9752 w9793 w9834 w9875 w9906 w9925 w10023 w10121 w10219 w10318 w10417 w10516 w10615 w10714 w10813 w10912 w11011 w11110 w11209 w11308 w11407 w11506 w11605 w11704 w11803 w11902 w12001 w12100 w12199 w12298 w12397 w12496 w12595 w12694 w12793 w12892 w12991 w13090 w13189 w13288 w13387 w13486 w13585 w13684 w13783 w13882 w13981 w14080 w14179 w14278 w14377 w14476 w14575 w14674 w14773 w14872 w14971 w15070 w15169 w15268 w15367 w15466 w15565 w15664 w15763]
      tunnel: [w288 w1240 w1252 w1265 w1284 w1416 w1453 w1493 w1518 w1534 w1545 w1556 w1571 w1586 w1601 w1616 w1639 w1659 w1683 w1715 w1769 w1814 w1836 w1858 w1873 w1907 w1925 w1943 w1962 w1993 w2028 w2047 w2073 w2106 w2129 w2147 w2181 w2201 w2224 w2262 w2282 w2314 w2359 w2390 w2445 w2499 w2575 w2650 w2725 w2800 w2875 w2936 w3039 w3095 w3189 w3273 w3355 w3437 w3519 w3601 w3683 w3765 w3847 w3929 w4011 w4093 w4176 w4259 w4342 w4425 w4508 w4573 w4692 w4775 w4858 w4941 w5025 w5109 w5193 w5277 w5361 w5445 w5529 w5613 w5697 w5781 w5866 w5951 w6036 w6121 w6206 w6291 w6376 w6461 w6546 w6631 w6717 w6803 w6889 w6975 w7061 w7147 w7233 w7319 w7405 w7456 w7497 w7538 w7579 w7620 w7661 w7702 w7743 w7784 w7825 w7866 w7907 w7948 w7989 w8030 w8071 w8112 w8153 w8194 w8235 w8276 w8317 w8358 w8399 w8440 w8481 w8522 w8563 w8604 w8645 w8686 w8727 w8768 w8809 w8850 w8891 w8932 w8973 w9014 w9055 w9096 w9137 w9178 w9219 w9260 w9301 w9342 w9383 w9424 w9465 w9506 w9547 w9588 w9629 w9670 w9711 w9752 w9793 w9834 w9875 w9906 w9925 w10023 w10121 w10219 w10318 w10417 w10516 w10615 w10714 w10813 w10912 w11011 w11110 w11209 w11308 w11407 w11506 w11605 w11704 w11803 w11902 w12001 w12100 w12199 w12298 w12397 w12496 w12595 w12694 w12793 w12892 w12991 w13090 w13189 w13288 w13387 w13486 w13585 w13684 w13783 w13882 w13981 w14080 w14179 w14278 w14377 w14476 w14575 w14674 w14773 w14872 w14971 w15070 w15169 w15268 w15367 w15466 w15565 w15664 w15763] -> w252
      tunnel: w251 -> [w287 w1239 w1251 w1264 w1283 w1415 w1452 w1492 w1517 w1533 w1544 w1555 w1570 w1585 w1600 w1615 w1638 w1658 w1682 w1714 w1768 w1810 w1833 w1855 w1874 w1906 w1922 w1942 w1961 w1992 w2027 w2046 w2072 w2105 w2128 w2146 w2180 w2200 w2223 w2261 w2281 w2313 w2358 w2389 w2444 w2498 w2574 w2649 w2724 w2799 w2874 w2935 w3038 w3114 w3188 w3272 w3354 w3436 w3518 w3600 w3682 w3764 w3846 w3928 w4010 w4092 w4175 w4258 w4341 w4424 w4507 w4572 w4691 w4774 w4857 w4940 w5024 w5108 w5192 w5276 w5360 w5444 w5528 w5612 w5696 w5780 w5865 w5950 w6035 w6120 w6205 w6290 w6375 w6460 w6545 w6630 w6716 w6802 w6888 w6974 w7060 w7146 w7232 w7318 w7404 w7455 w7496 w7537 w7578 w7619 w7660 w7701 w7742 w7783 w7824 w7865 w7906 w7947 w7988 w8029 w8070 w8111 w8152 w8193 w8234 w8275 w8316 w8357 w8398 w8439 w8480 w8521 w8562 w8603 w8644 w8685 w8726 w8767 w8808 w8849 w8890 w8931 w8972 w9013 w9054 w9095 w9136 w9177 w9218 w9259 w9300 w9341 w9382 w9423 w9464 w9505 w9546 w9587 w9628 w9669 w9710 w9751 w9792 w9833 w9874 w9905 w9924 w10022 w10120 w10218 w10317 w10416 w10515 w10614 w10713 w10812 w10911 w11010 w11109 w11208 w11307 w11406 w11505 w11604 w11703 w11802 w11901 w12000 w12099 w12198 w12297 w12396 w12495 w12594 w12693 w12792 w12891 w12990 w13089 w13188 w13287 w13386 w13485 w13584 w13683 w13782 w13881 w13980 w14079 w14178 w14277 w14376 w14475 w14574 w14673 w14772 w14871 w14970 w15069 w15168 w15267 w15366 w15465 w15564 w15663 w15762]
      tunnel: [w287 w1239 w1251 w1264 w1283 w1415 w1452 w1492 w1517 w1533 w1544 w1555 w1570 w1585 w1600 w1615 w1638 w1658 w1682 w1712 w1768 w1810 w1833 w1855 w1874 w1906 w1922 w1942 w1961 w1992 w2027 w2046 w2072 w2105 w2128 w2146 w2180 w2200 w2223 w2261 w2281 w2313 w2358 w2389 w2444 w2498 w2574 w2649 w2724 w2799 w2874 w2935 w3038 w3114 w3188 w3272 w3354 w3436 w3518 w3600 w3682 w3764 w3846 w3928 w4010 w4092 w4175 w4258 w4341 w4424 w4507 w4572 w4691 w4774 w4857 w4940 w5024 w5108 w5192 w5276 w5360 w5444 w5528 w5612 w5696 w5780 w5865 w5950 w6035 w6120 w6205 w6290 w6375 w6460 w6545 w6630 w6716 w6802 w6888 w6974 w7060 w7146 w7232 w7318 w7404 w7455 w7496 w7537 w7578 w7619 w7660 w7701 w7742 w7783 w7824 w7865 w7906 w7947 w7988 w8029 w8070 w8111 w8152 w8193 w8234 w8275 w8316 w8357 w8398 w8439 w8480 w8521 w8562 w8603 w8644 w8685 w8726 w8767 w8808 w8849 w8890 w8931 w8972 w9013 w9054 w9095 w9136 w9177 w9218 w9259 w9300 w9341 w9382 w9423 w9464 w9505 w9546 w9587 w9628 w9669 w9710 w9751 w9792 w9833 w9874 w9905 w9924 w10022 w10120 w10218 w10317 w10416 w10515 w10614 w10713 w10812 w10911 w11010 w11109 w11208 w11307 w11406 w11505 w11604 w11703 w11802 w11901 w12000 w12099 w12198 w12297 w12396 w12495 w12594 w12693 w12792 w12891 w12990 w13089 w13188 w13287 w13386 w13485 w13584 w13683 w13782 w13881 w13980 w14079 w14178 w14277 w14376 w14475 w14574 w14673 w14772 w14871 w14970 w15069 w15168 w15267 w15366 w15465 w15564 w15663 w15762] -> w250
      tunnel: w249 -> [w271 _ _ _ w1272 _ _ _ _ _ _ _ _ _ _ _ _ _ _ _ _ _ _ _ _ _ _ _ _ _ w2026 _ _ _ w2125 _ _ w2199 w2222 w2260 w2271 w2312 w2357 _ _ _ _ _ _ _ _ _ _ _ _ _ _ _ _ _ _ _ _ _ _ _ _ _ _ _ _ _ _ _ _ _ _ _ _ _ _ _ _ _ _ _ _ _ _ _ _ _ _ _ _ _ _ _ _ _ _ _ _ _ _ _ _ _ _ _ _ _ _ _ _ _ _ _ _ _ _ _ _ _ _ _ _ _ _ _ _ _ _ _ _ _ _ _ _ _ _ _ _ _ _ _ _ _ _ _ _ _ _ _ _ _ _ _ _ _ _ _ _ _ _ _ _ _ _ _ _ _ _ _ _ _ _ _ _ _ _ _ _ _ _ _ _ _ _ _ _ _ _ _ _ _ _ _ _ _ _ _ _ _ _ _ _ _ _ _ _ _ _ _ _ _ _ _ _ _ _ _ _ _ _ _]
      tunnel: w239 -> [w284 _ w1247 w1263 _ _ w1434 _ _ _ _ _ _ _ _ _ _ w1655 _ w1702 w1761 _ _ _ _ _ _ _ _ w1975 _ _ _ _ _ _ _ _ _ _ _ _ _ _ w2434 w2484 w2557 w2634 w2707 w2783 w2857 w2920 w3021 w3097 w3172 w3256 w3338 w3420 w3502 w3584 w3666 w3748 w3830 w3912 w3994 w4076 w4159 w4242 w4325 w4408 w4491 w4556 w4675 w4758 w4841 w4924 w5008 w5092 w5176 w5260 w5344 w5428 w5512 w5596 w5680 w5764 w5849 w5934 w6019 w6104 w6189 w6274 w6359 w6444 w6529 w6615 w6701 w6787 w6873 w6959 w7045 w7131 w7217 w7303 w7389 w7450 w7492 w7532 w7573 w7614 w7655 w7696 w7737 w7778 w7819 w7860 w7901 w7942 w7983 w8024 w8066 w8106 w8147 w8188 w8229 w8271 w8311 w8353 w8393 w8434 w8476 w8516 w8557 w8598 w8639 w8680 w8721 w8762 w8804 w8844 w8885 w8926 w8968 w9009 w9049 w9090 w9131 w9172 w9213 w9254 w9295 w9336 w9377 w9418 w9459 w9500 w9541 w9582 w9623 w9664 w9705 w9746 w9787 w9828 w9869 _ w9917 w10015 w10113 w10211 w10310 w10409 w10508 w10607 w10706 w10805 w10904 w11003 w11102 w11201 w11300 w11399 w11498 w11597 w11696 w11795 w11894 w11993 w12092 w12191 w12290 w12389 w12488 w12587 w12686 w12785 w12884 w12983 w13082 w13181 w13280 w13379 w13478 w13577 w13676 w13775 w13874 w13973 w14072 w14171 w14270 w14369 w14468 w14567 w14666 w14765 w14864 w14963 w15062 w15161 w15260 w15359 w15458 w15557 w15656 w15755]
      tunnel: [w283 w1238 w1250 w1261 w1276 w1408 w1451 w1491 w1516 w1532 w1543 w1554 w1569 w1584 w1599 w1614 w1632 w1657 w1681 w1711 w1767 w1804 w1826 w1849 w1872 w1905 w1923 w1940 w1958 w1990 w2019 w2045 w2071 w2104 w2123 w2145 w2178 w2197 w2220 w2258 w2280 w2310 w2355 w2388 w2443 w2494 w2569 w2645 w2719 w2794 w2869 w2930 w3033 w3109 w3184 w3267 w3349 w3431 w3513 w3595 w3677 w3759 w3841 w3923 w4005 w4087 w4170 w4253 w4336 w4419 w4502 w4567 w4686 w4769 w4852 w4935 w5019 w5103 w5187 w5271 w5355 w5439 w5523 w5607 w5691 w5775 w5860 w5945 w6030 w6115 w6200 w6285 w6370 w6455 w6540 w6625 w6711 w6797 w6883 w6969 w7055 w7141 w7227 w7313 w7399 w7454 w7495 w7536 w7577 w7618 w7659 w7700 w7741 w7782 w7823 w7864 w7905 w7946 w7987 w8028 w8069 w8110 w8151 w8192 w8233 w8274 w8315 w8356 w8397 w8438 w8479 w8520 w8561 w8602 w8643 w8684 w8725 w8766 w8807 w8848 w8889 w8930 w8971 w9012 w9053 w9094 w9135 w9176 w9217 w9258 w9299 w9340 w9381 w9422 w9463 w9504 w9545 w9586 w9627 w9668 w9709 w9750 w9791 w9832 w9873 w9904 w9923 w10021 w10119 w10217 w10316 w10415 w10514 w10613 w10712 w10811 w10910 w11009 w11108 w11207 w11306 w11405 w11504 w11603 w11702 w11801 w11900 w11999 w12098 w12197 w12296 w12395 w12494 w12593 w12692 w12791 w12890 w12989 w13088 w13187 w13286 w13385 w13484 w13583 w13682 w13781 w13880 w13979 w14078 w14177 w14276 w14375 w14474 w14573 w14672 w14771 w14870 w14969 w15068 w15167 w15266 w15365 w15464 w15563 w15662 w15761] -> w248
      tunnel: w247 -> [w282 w1238 w1250 w1261 w1276 w1408 w1451 w1491 w1516 w1532 w1543 w1554 w1569 w1584 w1599 w1614 w1632 w1657 w1681 w1711 w1767 w1804 w1826 w1849 w1872 w1905 w1923 w1940 w1958 w1990 w2019 w2045 w2071 w2104 w2123 w2145 w2178 w2197 w2220 w2258 w2280 w2310 w2355 w2388 w2443 w2494 w2569 w2645 w2719 w2794 w2869 w2930 w3033 w3109 w3184 w3267 w3349 w3431 w3513 w3595 w3677 w3759 w3841 w3923 w4005 w4087 w4170 w4253 w4336 w4419 w4502 w4567 w4686 w4769 w4852 w4935 w5019 w5103 w5187 w5271 w5355 w5439 w5523 w5607 w5691 w5775 w5860 w5945 w6030 w6115 w6200 w6285 w6370 w6455 w6540 w6625 w6711 w6797 w6883 w6969 w7055 w7141 w7227 w7313 w7399 w7454 w7495 w7536 w7577 w7618 w7659 w7700 w7741 w7782 w7823 w7864 w7905 w7946 w7987 w8028 w8069 w8110 w8151 w8192 w8233 w8274 w8315 w8356 w8397 w8438 w8479 w8520 w8561 w8602 w8643 w8684 w8725 w8766 w8807 w8848 w8889 w8930 w8971 w9012 w9053 w9094 w9135 w9176 w9217 w9258 w9299 w9340 w9381 w9422 w9463 w9504 w9545 w9586 w9627 w9668 w9709 w9750 w9791 w9832 w9873 w9904 w9923 w10021 w10119 w10217 w10316 w10415 w10514 w10613 w10712 w10811 w10910 w11009 w11108 w11207 w11306 w11405 w11504 w11603 w11702 w11801 w11900 w11999 w12098 w12197 w12296 w12395 w12494 w12593 w12692 w12791 w12890 w12989 w13088 w13187 w13286 w13385 w13484 w13583 w13682 w13781 w13880 w13979 w14078 w14177 w14276 w14375 w14474 w14573 w14672 w14771 w14870 w14969 w15068 w15167 w15266 w15365 w15464 w15563 w15662 w15761]
